vi "Convert Package Attribute String to Cluster.vi"(8 "error in (no error)":errorcluster, 11 "package attributes string":string) -> (0 "error out":errorcluster, 3 "package attributes":T1={"Package Name"="", "Display name"="", "Version"="", "Display version"="", "Synopsis"="", "Description"="", "Maintainer"="", "Maintainer email address"="", "Category"="", "Homepage"="", "Release notes"="", "Depends"=[], "Recommends"=[], "Suggests"=[], "Conflicts"=[], "Provides"=[], "Replaces"=[], "Supplements"=[], "Enhances"=[], "Product"=FALSE, "User visible"=FALSE, "Installed size (KB)"=0, "Package filesize (bytes)"=0, "Architecture"="", "Agent"="file", "MD5Checksum"=""})   [LabVIEW 2014, in "NIPM_API.lvlib"]
doc: "Converts a package attribute string to a package attribute cluster\n\nINPUT(s)\n<B>package attributes string</B>: This is the string containing the package attributes and values. For example, this string could come from the output of a nipkg CLI command.\n\nOUTPUT(s)\n<B>Package attributes</B>: Returns a cluster of package attributes"
uses:
  NIPM_API.lvlib
  package attributes.ctl
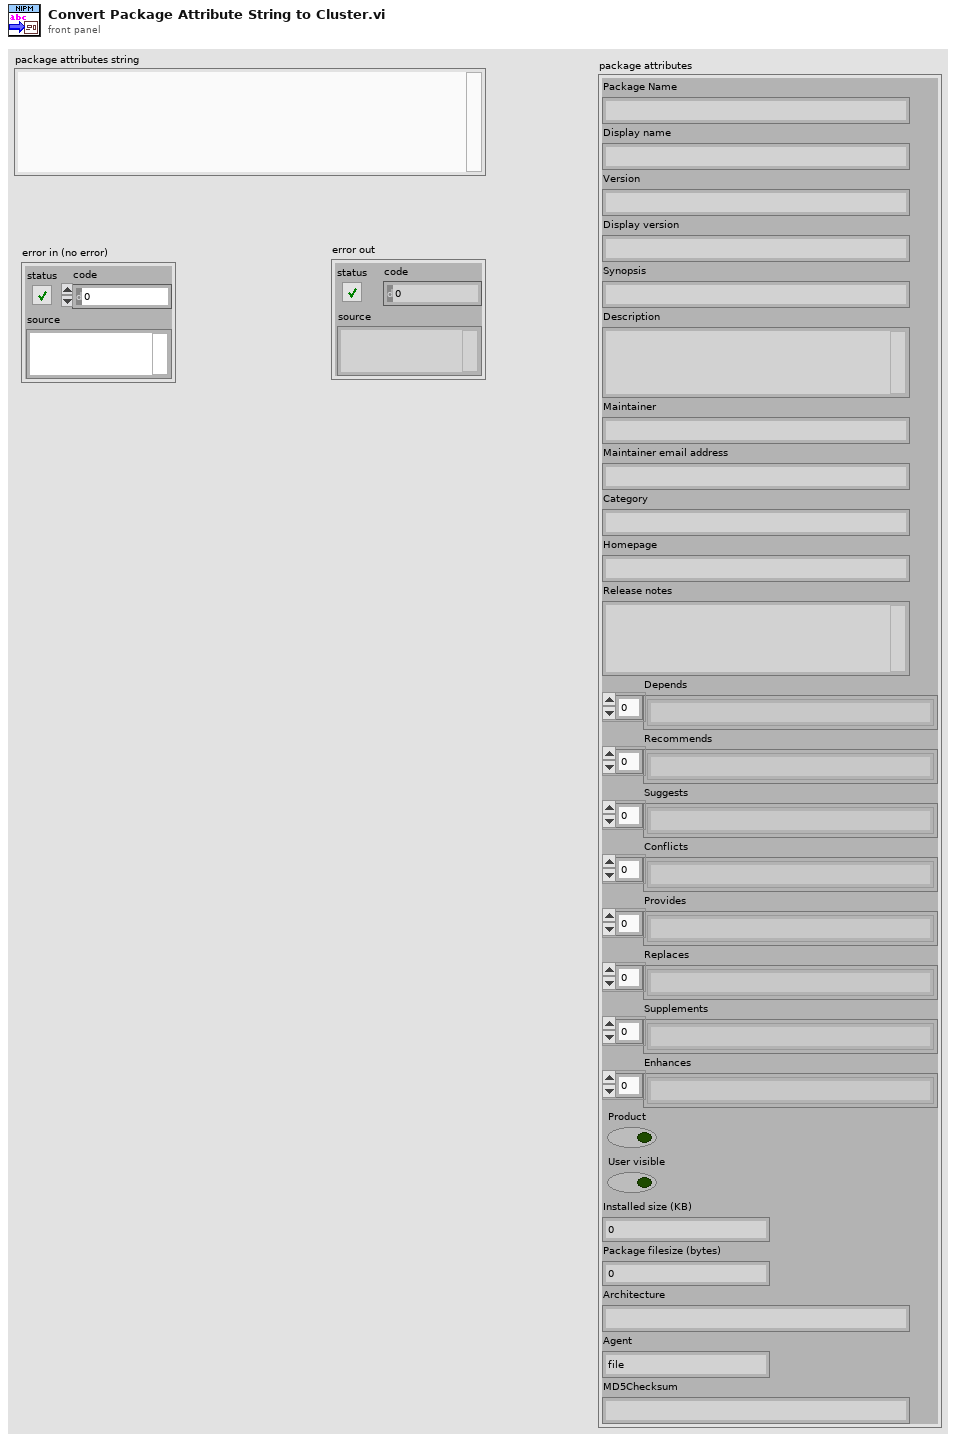
[diagram p1: front panel]
types:
  T1 = typedef "NIPM_API.lvlib/package attributes.ctl" = cluster{"Package Name":string, "Display name":string, "Version":string, "Display version":string, "Synopsis":string, "Description":string, "Maintainer":string, "Maintainer email address":string, "Category":string, "Homepage":string, "Release notes":string, "Depends":string[], "Recommends":string[], "Suggests":string[], "Conflicts":string[], "Provides":string[], "Replaces":string[], "Supplements":string[], "Enhances":string[], "Product":bool, "User visible":bool, "Installed size (KB)":u64, "Package filesize (bytes)":u64, "Architecture":string, "Agent":string, "MD5Checksum":string}
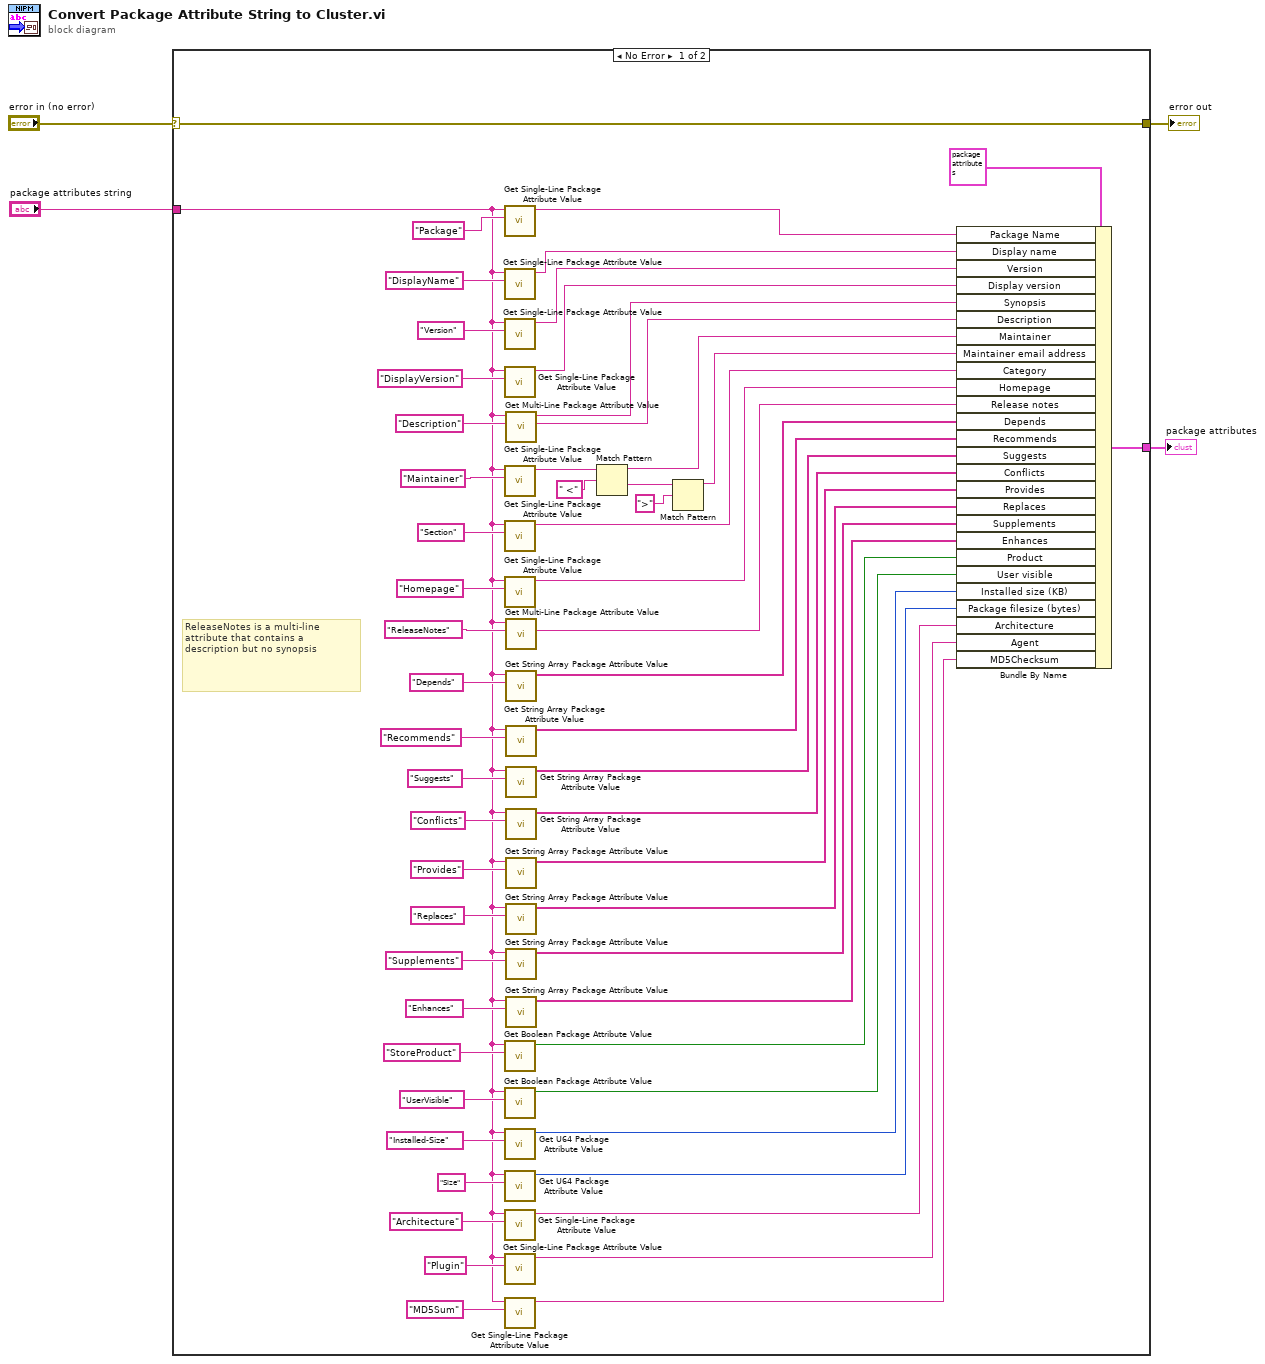
[diagram p0: block diagram]
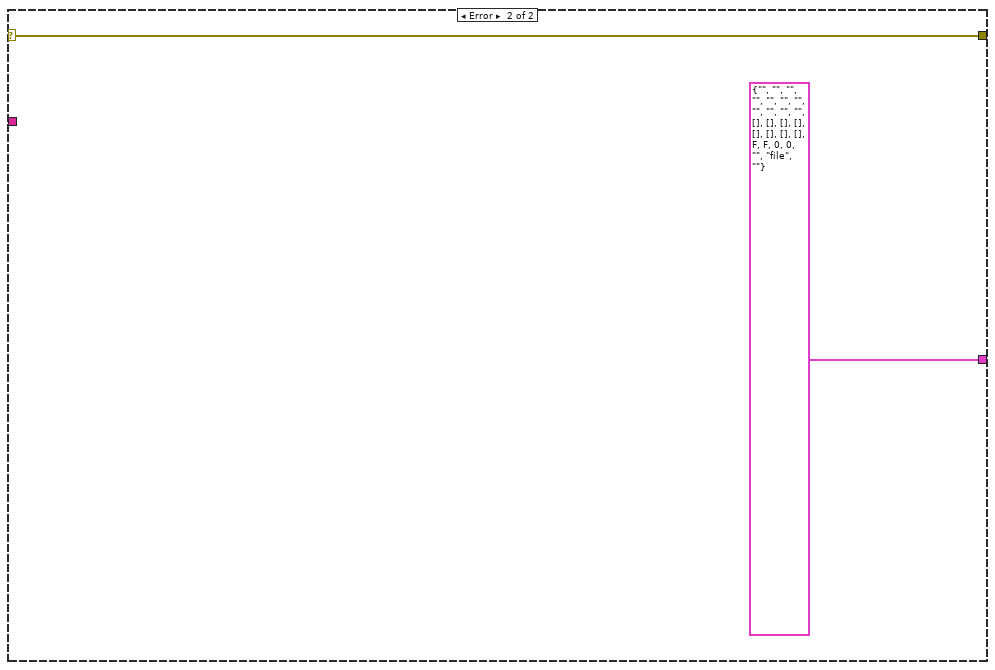
[diagram p2: hidden frame]
diagram:
  n1 = case shown="No Error" "error in (no error)" {
    selector: "error in (no error)" -> [w8 w64]
    tunnel: [w10 T1 {"Package Name"="", "Display name"="", "Version"="", "Display version"="", "Synopsis"="", "Description"="", "Maintainer"="", "Maintainer email address"="", "Category"="", "Homepage"="", "Release notes"="", "Depends"=[], "Recommends"=[], "Suggests"=[], "Conflicts"=[], "Provides"=[], "Replaces"=[], "Supplements"=[], "Enhances"=[], "Product"=FALSE, "User visible"=FALSE, "Installed size (KB)"=0, "Package filesize (bytes)"=0, "Architecture"="", "Agent"="file", "MD5Checksum"=""} ("package attributes")] -> w4
    tunnel: "package attributes string" -> [w9 _]
    tunnel: [w8 w64] -> w1
    frame No Error {
      # "ReleaseNotes is a multi-line attribute that contains a description but no synopsis"
      n2 = call "Get Single-Line Package Attribute Value.vi"("package attribute name"="Package" ("regular expression"), "package attributes CLI string"=w9) -> ("package attribute value"=w60:string)  [unwired: 7 in, 2 out]
      n3 = call "Get Single-Line Package Attribute Value.vi"("package attribute name"="DisplayName" ("Package Attribute Name"), "package attributes CLI string"=w9) -> ("package attribute value"=w58:string)  [unwired: 7 in, 2 out]
      n4 = call "Get Single-Line Package Attribute Value.vi"("package attribute name"="Version" ("Package Attribute Name"), "package attributes CLI string"=w9) -> ("package attribute value"=w55:string)  [unwired: 7 in, 2 out]
      n5 = call "Get Single-Line Package Attribute Value.vi"("package attribute name"="DisplayVersion" ("Package Attribute Name"), "package attributes CLI string"=w9) -> ("package attribute value"=w54:string)  [unwired: 7 in, 2 out]
      n6 = call "Get Single-Line Package Attribute Value.vi"("package attribute name"="Maintainer" ("Package Attribute Name"), "package attributes CLI string"=w9) -> ("package attribute value"=w44:string)  [unwired: 7 in, 2 out]
      n7 = call "Get Single-Line Package Attribute Value.vi"("package attribute name"="Section" ("Package Attribute Name"), "package attributes CLI string"=w9) -> ("package attribute value"=w50:string)  [unwired: 7 in, 2 out]
      n8 = call "Get Single-Line Package Attribute Value.vi"("package attribute name"="Homepage" ("Package Attribute Name"), "package attributes CLI string"=w9) -> ("package attribute value"=w48:string)  [unwired: 7 in, 2 out]
      n9 = call "Get Boolean Package Attribute Value.vi"("package attribute name"="StoreProduct" ("Package Attribute Name"), "package attributes CLI string"=w9) -> ("package attribute value"=w22:bool)  [unwired: 7 in, 2 out]
      n10 = call "Get Boolean Package Attribute Value.vi"("package attribute name"="UserVisible" ("Package Attribute Name"), "package attributes CLI string"=w9) -> ("package attribute value"=w21:bool)  [unwired: 7 in, 2 out]
      n11 = call "Get U64 Package Attribute Value.vi"("package attribute name"="Installed-Size" ("Package Attribute Name"), "package attributes CLI string"=w9) -> ("package attribute value"=w15:u64)  [unwired: 7 in, 2 out]
      n12 = call "Get U64 Package Attribute Value.vi"("package attribute name"="Size" ("Package Attribute Name"), "package attributes CLI string"=w9) -> ("package attribute value"=w13:u64)  [unwired: 7 in, 2 out]
      n13 = call "Get Single-Line Package Attribute Value.vi"("package attribute name"="Architecture" ("Package Attribute Name"), "package attributes CLI string"=w9) -> ("package attribute value"=w17:string)  [unwired: 7 in, 2 out]
      n14 = call "Get Single-Line Package Attribute Value.vi"("package attribute name"="Plugin" ("Package Attribute Name"), "package attributes CLI string"=w9) -> ("package attribute value"=w16:string)  [unwired: 7 in, 2 out]
      n15 = call "Get Single-Line Package Attribute Value.vi"("package attribute name"="MD5Sum" ("Package Attribute Name"), "package attributes CLI string"=w9) -> ("package attribute value"=w11:string)  [unwired: 7 in, 2 out]
      n16 = call "Get Multi-Line Package Attribute Value.vi"("package attribute name"="Description" ("Package Attribute Name"), "package attributes CLI string"=w9) -> ("description"=w6:string, "synopsis"=w7:string)  [unwired: 6 in, 2 out]
      n17 = call "Get Multi-Line Package Attribute Value.vi"("package attribute name"="ReleaseNotes" ("Package Attribute Name"), "package attributes CLI string"=w9) -> ("description"=w5:string)  [unwired: 6 in, 3 out]
      n18 = call "Get String Array Package Attribute Value.vi"("package attribute name"="Depends" ("Package Attribute Name"), "package attributes CLI string"=w9) -> ("package attribute value"=w39:string[])  [unwired: 7 in, 2 out]
      n19 = call "Get String Array Package Attribute Value.vi"("package attribute name"="Recommends" ("Package Attribute Name"), "package attributes CLI string"=w9) -> ("package attribute value"=w33:string[])  [unwired: 7 in, 2 out]
      n20 = call "Get String Array Package Attribute Value.vi"("package attribute name"="Suggests" ("Package Attribute Name"), "package attributes CLI string"=w9) -> ("package attribute value"=w32:string[])  [unwired: 7 in, 2 out]
      n21 = call "Get String Array Package Attribute Value.vi"("package attribute name"="Conflicts" ("Package Attribute Name"), "package attributes CLI string"=w9) -> ("package attribute value"=w31:string[])  [unwired: 7 in, 2 out]
      n22 = call "Get String Array Package Attribute Value.vi"("package attribute name"="Provides" ("Package Attribute Name"), "package attributes CLI string"=w9) -> ("package attribute value"=w30:string[])  [unwired: 7 in, 2 out]
      n23 = call "Get String Array Package Attribute Value.vi"("package attribute name"="Replaces" ("Package Attribute Name"), "package attributes CLI string"=w9) -> ("package attribute value"=w29:string[])  [unwired: 7 in, 2 out]
      n24 = call "Get String Array Package Attribute Value.vi"("package attribute name"="Supplements" ("Package Attribute Name"), "package attributes CLI string"=w9) -> ("package attribute value"=w26:string[])  [unwired: 7 in, 2 out]
      n25 = call "Get String Array Package Attribute Value.vi"("package attribute name"="Enhances" ("Package Attribute Name"), "package attributes CLI string"=w9) -> ("package attribute value"=w25:string[])  [unwired: 7 in, 2 out]
      n26 = Match Pattern(string=w44, regular expression=" <" ("Package Attribute Value")) -> (before substring=w45:string, after substring=w43:string)  [unwired: 1 in, 2 out]
      n27 = Match Pattern(string=w43, regular expression=">") -> (before substring=w41:string)  [unwired: 1 in, 3 out]
      n28 = Bundle By Name(cluster=T1 {"Package Name"="", "Display name"="", "Version"="", "Display version"="", "Synopsis"="", "Description"="", "Maintainer"="", "Maintainer email address"="", "Category"="", "Homepage"="", "Release notes"="", "Depends"=[], "Recommends"=[], "Suggests"=[], "Conflicts"=[], "Provides"=[], "Replaces"=[], "Supplements"=[], "Enhances"=[], "Product"=FALSE, "User visible"=FALSE, "Installed size (KB)"=0, "Package filesize (bytes)"=0, "Architecture"="", "Agent"="file", "MD5Checksum"=""} ("package attributes"), "Package Name"=w60, "Display name"=w58, "Version"=w55, "Display version"=w54, "Synopsis"=w7, "Description"=w6, "Maintainer"=w45, "Maintainer email address"=w41, "Category"=w50, "Homepage"=w48, "Release notes"=w5, "Depends"=w39, "Recommends"=w33, "Suggests"=w32, "Conflicts"=w31, "Provides"=w30, "Replaces"=w29, "Supplements"=w26, "Enhances"=w25, "Product"=w22, "User visible"=w21, "Installed size (KB)"=w15, "Package filesize (bytes)"=w13, "Architecture"=w17, "Agent"=w16, "MD5Checksum"=w11) -> (w10:T1)
    }
    frame Error {
    }
  }
  "package attributes" <- w4
  "error out" <- w1
